vi "ResetGyro.vi"   [LabVIEW 2013]
types:
  T1 = typedef "WPI_GyroDevRef.ctl" = cluster{"DevStatus":errorcluster, "Analog Module":T2, "Analog Channel":T3, "Offset":dbl, "Gain (VoltsPerDegree/Second)":dbl}
  T2 = typedef "FPGA_TypedefAnalogModule.ctl" = enum16{"Analog Module 1", "Analog Module 2"}
  T3 = typedef "FPGA_AIChannel.ctl" = enum8{"AI 1", "AI 2", "AI 3", "AI 4", "AI 5", "AI 6", "AI 7", "AI 8", "Invalid"}
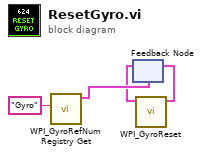
[diagram p0: block diagram]
diagram:
  n1 = call <vilib>:"WPI_GyroRefNum Registry Get.vi"("refnum name"="Gyro") -> ("GyroDevRef"=w3:T1)  [unwired: 9 in, 1 out]
  n2 = feedback #1(w3) -> (w2:T1)
  n3 = call <vilib>:"WPI_GyroReset.vi"("GyroDevRef"=w2) -> ("GyroDevRef"=w1:T1)  [unwired: 9 in, 1 out]
  n4 = feedback-in #1(w1) -> ()
